vi "Create Topic.vi"(8 "error in (no error)":errorcluster, 9 "Region":T1, 10 "Name":string, 11 "AWS Credentials":T2) -> (0 "error out":errorcluster, 3 "Topic out":refnum<class "Topic.lvclass">)   [LabVIEW 2015, in "NI_AWS_SNS.lvlib" / "Topic.lvclass"]
uses:
  Topic.lvclass
  Core/HTTP Request/AWS Credentials.ctl
  Core/HTTP Request/Region.ctl
  Core/HTTP Request/Name Value Pair.ctl
  Core/HTTP Request/Request Options.ctl
  Core/HTTP Request/Region handling.ctl
  Core/HTTP Request/URL formatting.ctl
  Core/HTTP Request/HTTP Request.lvclass
  Core/ARN/ARN.lvclass
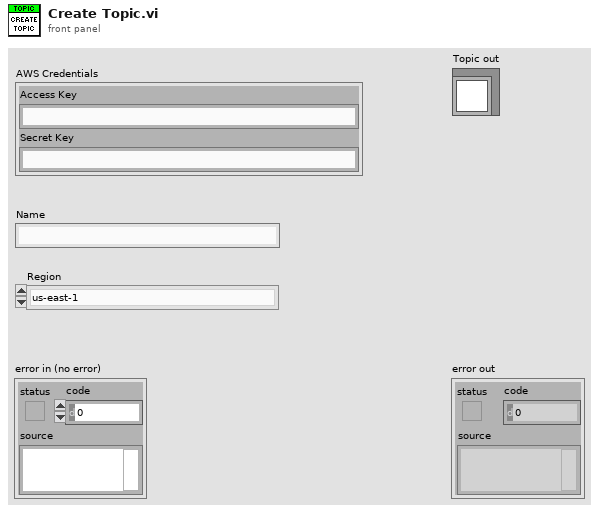
[diagram p1: front panel]
types:
  T1 = typedef "NI_AWS_Core.lvlib/HTTP Request.lvclass/Region.ctl" = enum16{"us-east-1", "us-east-2", "us-west-1", "us-west-2", "ap-northeast-1", "ap-northeast-2", "ap-southeast-1", "ap-southeast-2", "ca-central-1", "eu-central-1", "eu-west-1", "eu-west-2", "sa-east-1"}
  T2 = typedef "NI_AWS_Core.lvlib/HTTP Request.lvclass/AWS Credentials.ctl" = cluster{"Access Key":string, "Secret Key":string}
  T3 = typedef "NI_AWS_Core.lvlib/HTTP Request.lvclass/Request Options.ctl" = cluster{"request headers":T4[], "request parameters":T4[], "request body":string, "region handling":T5, "URL formatting":T6}
  T4 = typedef "NI_AWS_Core.lvlib/HTTP Request.lvclass/Name Value Pair.ctl" = cluster{"name":string, "value":string}
  T5 = typedef "NI_AWS_Core.lvlib/HTTP Request.lvclass/Region handling.ctl" = enum16{"use region everywhere", "use region (authentication only)", "use region (URL only)", "ignore region everwhere"}
  T6 = typedef "NI_AWS_Core.lvlib/HTTP Request.lvclass/URL formatting.ctl" = enum16{"region-", "region."}
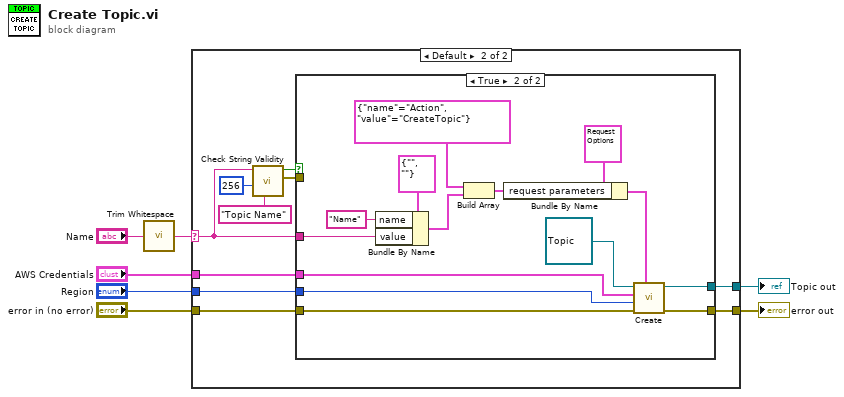
[diagram p0: block diagram]
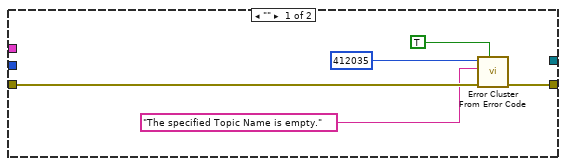
[diagram p2: hidden frame]
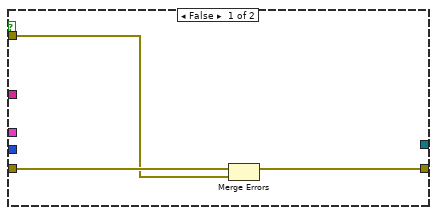
[diagram p3: hidden frame]
diagram:
  n1 = call <vilib>:"Trim Whitespace.vi"("string"="Name") -> ("trimmed string"=w1:string)  [unwired: 1 in]
  n2 = case shown="Default" w1 {
    selector: w1 -> [_ w17]
    tunnel: [_ w22] -> w6
    tunnel: [w11 w21] -> w5
    tunnel: "error in (no error)" -> [w12 w20]
    tunnel: "AWS Credentials" -> [_ w19]
    tunnel: "Region" -> [_ w18]
    frame "" {
      n3 = call <vilib>:"Error Cluster From Error Code.vi"("show call chain? (False)"=TRUE, "error in (no error)"=w12, "error message (\"\")"="The specified Topic Name is empty.", "error code (0)"=412035) -> ("error out"=w11:errorcluster)  [unwired: 5 in]
    }
    frame Default {
      n4 = call "Check String Validity.vi"("String Name for Error"="Topic Name", "Max Characters"=256, "String"=w17) -> ("string error"=w15:errorcluster, "Valid"=w16:bool)  [unwired: 7 in]
      n5 = case shown="True" w16 {
        tunnel: [_ w32] -> w22
        tunnel: [w24 w30] -> w21
        tunnel: w20 -> [w25 w29]
        tunnel: w19 -> [_ w28]
        tunnel: w18 -> [_ w27]
        tunnel: w17 -> [_ w26]
        tunnel: w15 -> [w23 _]
        frame False {
          n6 = Merge Errors(w25, w23) -> (w24:errorcluster)
        }
        frame True {
          n7 = Bundle By Name(cluster=T4 {"name"="", "value"=""} ("element"), "name"="Name", "value"=w26) -> (w39:T4)
          n8 = Build Array(T4 {"name"="Action", "value"="CreateTopic"} ("Name Value Pair"), w39) -> (w35:T4[])
          n9 = Bundle By Name(cluster=T3 {"request headers"=[], "request parameters"=[{"name"="Action", "value"="ListQueues"}], "request body"="", "region handling"=enum."use region everywhere", "URL formatting"=enum."region."} ("Request Options"), "request parameters"=w35) -> (w31:T3)
          n10 = call "Create.vi"("Request Options"=w31, "error in (no error)"=w29, "Region"=w27, "AWS Credentials"=w28, "ARN in"=refnum<class "Topic.lvclass"> refnum ("NI_SNS.lvclass")) -> ("error out"=w30:errorcluster, "ARN out"=w32:refnum<class "Topic.lvclass">)  [unwired: 5 in]
        }
      }
    }
  }
  "error out" <- w5
  "Topic out" <- w6
